vi "HexToWord.vi"(11 "数组":u16[](array[numeric]) format="%04xH") -> (3 "WORD":u16[](array[numeric]))   [LabVIEW 2016, in "环境动力监测库.lvlib"]
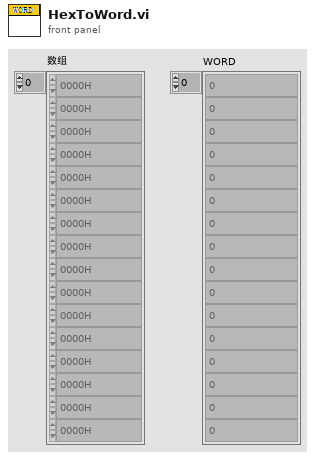
[diagram p1: front panel]
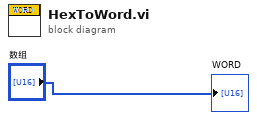
[diagram p0: block diagram]
diagram:
  "WORD" <- "数组"
